vi "Simple Plotter.vi"() -> ()   [LabVIEW 2012]
uses:
  <vilib>/Analysis/NI_AALBase.lvlib
  <vilib>/Analysis/baseanly.llb/Mean (DBL).vi
panel:
  out "Mean":dbl format="%0.2f"
  out "Current Mean":dbl
  out "Current Temperature":dbl
  out "Min value":dbl
  out "Max value":dbl
  in  "Stop Button":bool
  out "History":dbl(graph)
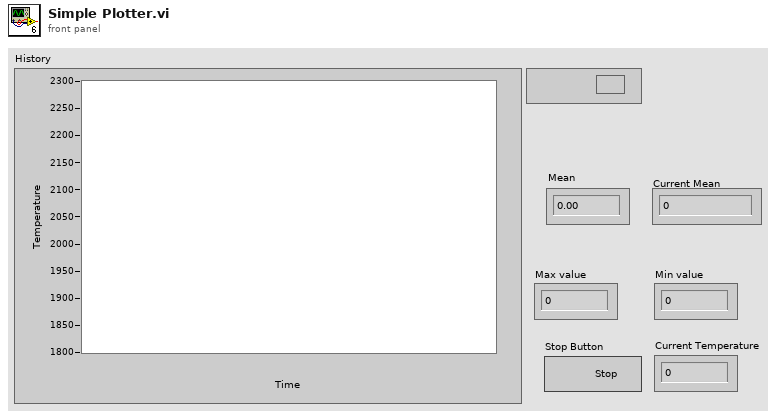
[diagram p1: front panel]
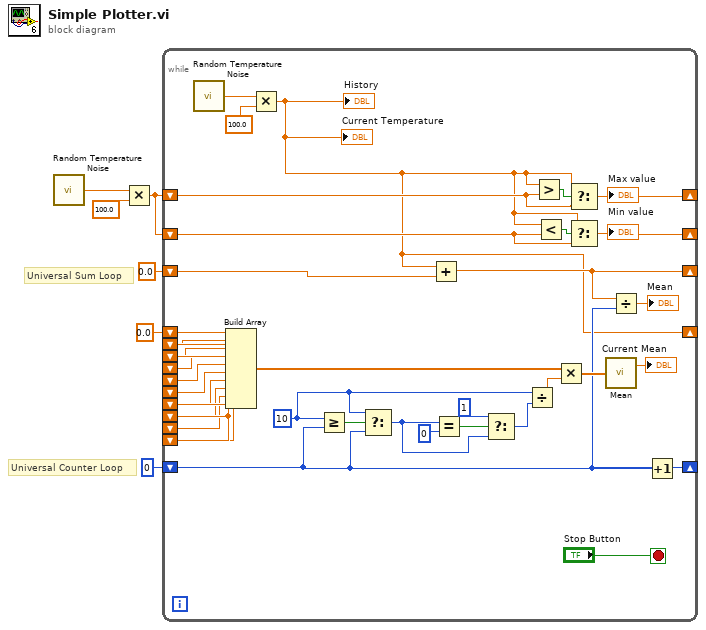
[diagram p0: block diagram]
diagram:
  w1 = 0.0
  # "Universal Sum Loop"
  # "Universal Counter Loop"
  n1 = call "Random Temperature Noise.vi"() -> ("Temperature"=w5:dbl)  [unwired: 1 in]
  n2 = Multiply(x=w5, y=100.0) -> (x*y=w3:dbl)
  n3 = while {
    shift-right: [w21] -> _
    shift-left: 0.0 -> [w20]
    shift-right: [w37] -> _
    shift-left: w3 -> [w35]
    shift-right: [w36] -> _
    shift-left: w3 -> [w34]
    shift-right: [w7] -> _
    shift-left: w1 -> [w31]
    shift-left: w1 -> [w30]
    shift-left: w1 -> [w22]
    shift-left: w1 -> [w29]
    shift-left: w1 -> [w24]
    shift-left: w1 -> [w25]
    shift-right: [w32] -> _
    shift-left: 0 -> [w8]
    shift-left: w1 -> [w23]
    shift-left: w1 -> [w28]
    shift-left: w1 -> [w26]
    shift-left: w1 -> [w27]
    stop <- "Stop Button" stop-if-true
    w15 = u8 10 ("y")
    n4 = call "Random Temperature Noise.vi"() -> ("Temperature"=w40:dbl)  [unwired: 1 in]
    n5 = Build Array(w31, w30, w29, w28, w27, w26, w25, w24, w23, w22) -> (w12:dbl[])
    n6 = Multiply(x=w40, y=100.0) -> (x*y=w7:dbl)
    "History" <- w7
    "Current Temperature" <- w7
    n7 = Greater Or Equal?(x=w15, y=w8) -> (x >= y?=w16:bool)
    n8 = Select(t=w15, s=w16, f=w8) -> (s? t:f=w14:i32)
    n9 = Add(x=w7, y=w20) -> (x+y=w21:dbl)
    n10 = Equal?(x=w14, y=u8 0) -> (x = y?=w17:bool)
    n11 = Select(t=1, s=w17, f=w14) -> (s? t:f=w9:i32)
    n12 = Divide(x=w15, y=w9) -> (x/y=w13:dbl)
    n13 = Greater?(x=w7, y=w35) -> (0:w39:bool)
    n14 = Less?(x=w7, y=w34) -> (x < y?=w38:bool)
    n15 = Multiply(x=w12, y=w13) -> (x*y=w11:dbl[])
    n16 = Select(t=w7, s=w39, f=w35) -> (s? t:f=w37:dbl)
    "Max value" <- w37
    n17 = Select(t=w7, s=w38, f=w34) -> (s? t:f=w36:dbl)
    "Min value" <- w36
    n18 = call-poly <vilib>:"Mean.vi"("X"=w11) -> ("mean"=→"Current Mean":dbl)  [unwired: 1 out]
    n19 = Divide(x=w21, y=w8) -> (x/y=→"Mean":dbl)
    n20 = Increment(x=w8) -> (x+1=w32:i32)
  }
